vi "vi_Gen_Test_Single_Cell.vi"() -> ()   [LabVIEW 2025]
panel:
  in  "Output Safety":T1
  in  "filepath":path
  in  "Batteryname":string
  in  "Starting Cycle":i32
  out "PS error out":errorcluster
  out "PS VIS resource name out":refnum<visa-resource-name>
  in  "Charge Current Cutoff":dbl
  in  "Charge Current Setpoint 2":dbl format="%#.6g"
  in  "charge Voltage Setpoint  2":dbl format="%#.6g"
  in  "Wait time":dbl
  in  "Discharge Current Cutoff":dbl
  in  "Discharge Current Setpoint":dbl format="%#.6g"
  in  "Discharge Voltage Setpoint":dbl format="%#.6g"
  in  "NHR VISA":refnum<visa-resource-name>
  in  "NHR error in":errorcluster
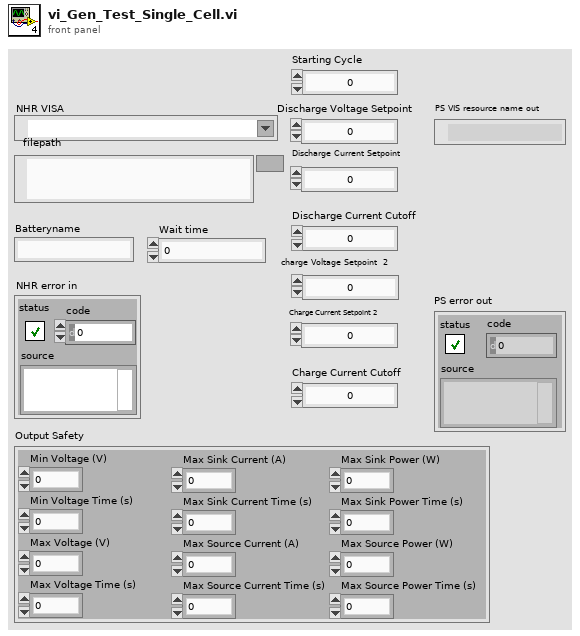
[diagram p1: front panel]
types:
  T1 = cluster{"Min Voltage (V)":dbl, "Min Voltage Time (s)":dbl, "Max Voltage (V)":dbl, "Max Voltage Time (s)":dbl, "Max Sink Current (A)":dbl, "Max Sink Current Time (s)":dbl, "Max Source Current (A)":dbl, "Max Source Current Time (s)":dbl, "Max Sink Power (W)":dbl, "Max Sink Power Time (s)":dbl, "Max Source Power (W)":dbl, "Max Source Power Time (s)":dbl}
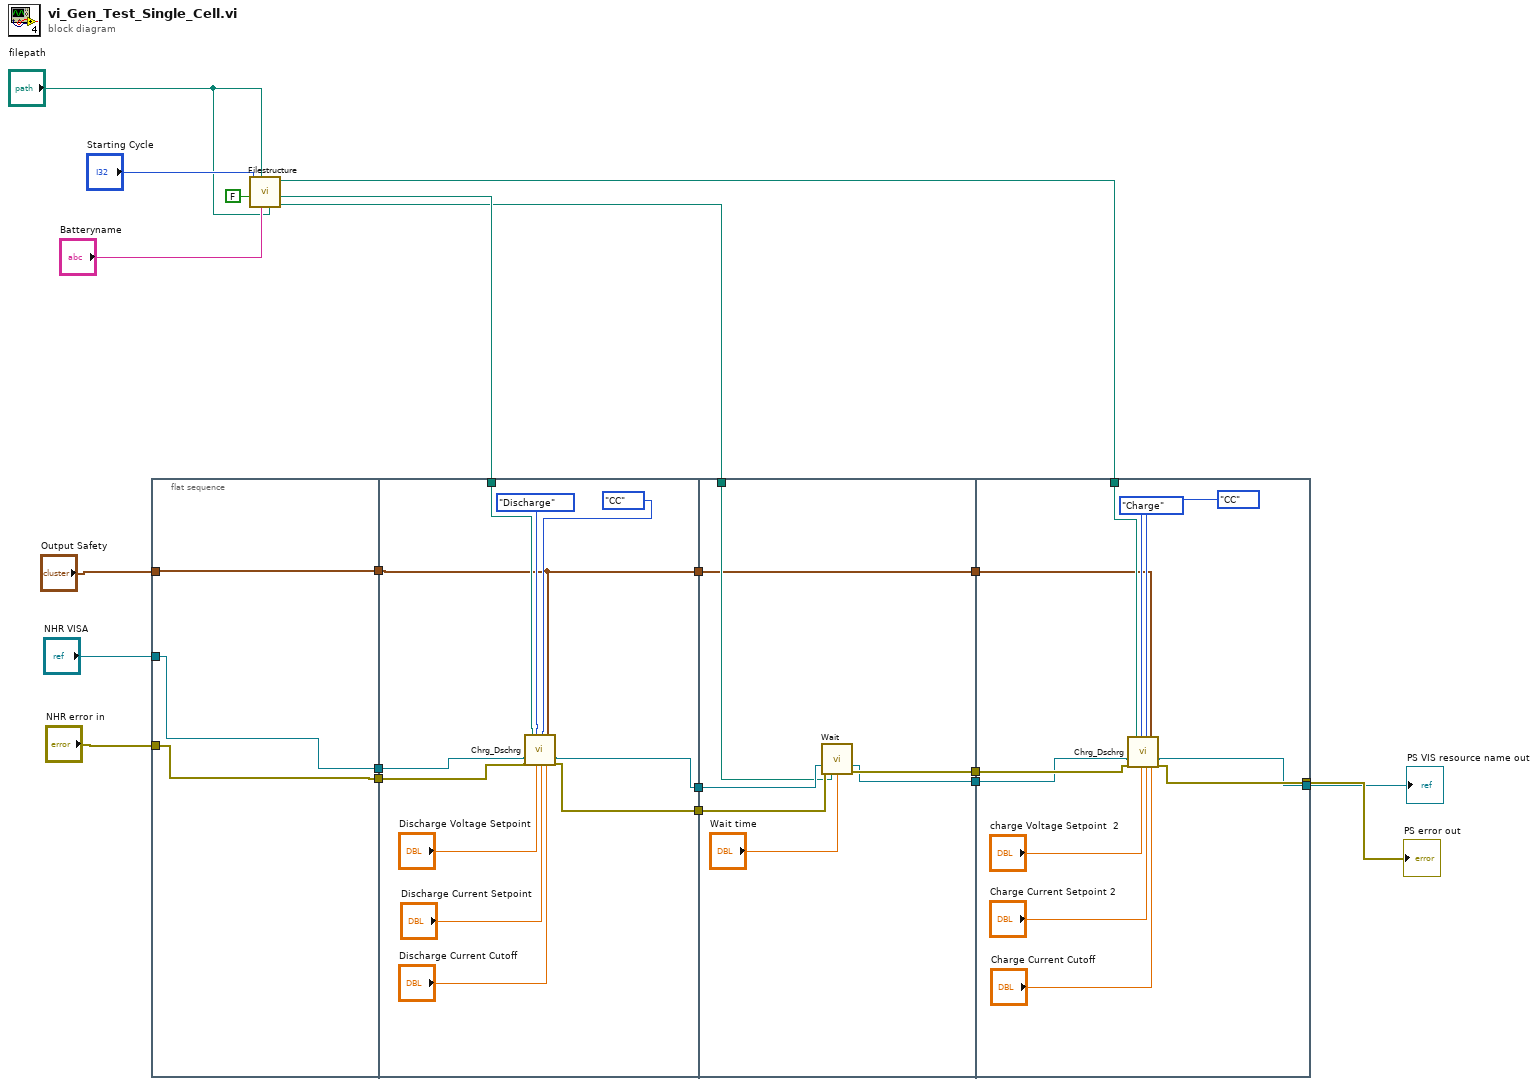
[diagram p0: block diagram]
diagram:
  n1 = flat-sequence {
    tunnel: "NHR error in" -> [w23]
    tunnel: "NHR VISA" -> [w24]
    tunnel: [w24] -> w19
    tunnel: [w23] -> w18
    tunnel: "Output Safety" -> [w22]
    tunnel: [w22] -> w4
    tunnel: w19 -> [w29]
    tunnel: w18 -> [w30]
    tunnel: [w35] -> w17
    tunnel: [w34] -> w16
    tunnel: w8 -> [w28]
    tunnel: w4 -> [w25]
    tunnel: [w25] -> w3
    tunnel: w17 -> [w42]
    tunnel: w16 -> [w41]
    tunnel: [w39] -> w15
    tunnel: [w38] -> w14
    tunnel: w7 -> [w37]
    tunnel: w3 -> [w36]
    tunnel: [w36] -> w2
    tunnel: w15 -> [w50]
    tunnel: w14 -> [w49]
    tunnel: [w44] -> w13
    tunnel: [w43] -> w12
    tunnel: w6 -> [w48]
    tunnel: w2 -> [w45]
    frame #0 {
    }
    frame #1 {
      n2 = call "Chrg_Dschrg.vi"("PS VISA in"=w29, "PS error in"=w30, "DischargeCyclePath"=w28, "Charge/discharge"=enum8{"Charge", "Discharge"}."Discharge", "Charge/Discharge Voltage Setpoint"="Discharge Voltage Setpoint", "CC or CCCV"=enum16{"CC", "CCCV"}."CC", "Current Setpoint"="Discharge Current Setpoint", "Output Safety"=w25, "Current Cutoff"="Discharge Current Cutoff") -> ("PS VIS resource name out"=w35:refnum<visa-resource-name>, "PS error out"=w34:errorcluster)  [unwired: 9 in]
    }
    frame #2 {
      n3 = call "Wait.vi"("PS VISA in"=w42, "PS error in"=w41, "Wait Filepath"=w37, "Wait time"="Wait time") -> ("PS Visa Out"=w38:refnum<visa-resource-name>, "PS error out"=w39:errorcluster)  [unwired: 10 in]
    }
    frame #3 {
      n4 = call "Chrg_Dschrg.vi"("PS VISA in"=w49, "PS error in"=w50, "DischargeCyclePath"=w48, "Charge/discharge"=enum8{"Charge", "Discharge"}."Charge", "Charge/Discharge Voltage Setpoint"="charge Voltage Setpoint  2", "CC or CCCV"=enum16{"CC", "CCCV"}."CC", "Current Setpoint"="Charge Current Setpoint 2", "Output Safety"=w45, "Current Cutoff"="Charge Current Cutoff") -> ("PS VIS resource name out"=w43:refnum<visa-resource-name>, "PS error out"=w44:errorcluster)  [unwired: 9 in]
    }
  }
  n5 = call "Filestructure.vi"("Discharge filepath"="filepath", "Batteryname"="Batteryname", "Charge filepath"="filepath", "In for loop"=FALSE, "Starting Cycle"="Starting Cycle") -> ("DischargeWaitPath"=w7:path, "DischargeCyclePath"=w8:path, "ChargeCyclePath"=w6:path)  [unwired: 2 in, 2 out]
  "PS error out" <- w13
  "PS VIS resource name out" <- w12
